vi "GetTempConfigByName.vi"(3 "Error In":errorcluster, 4 "JSON":string, 5 "Name":string) -> (0 "Error Out":errorcluster, 1 "Exist":bool, 2 "TempConfig":T1)   [LabVIEW 2014]
uses:
  TempConfig.ctl
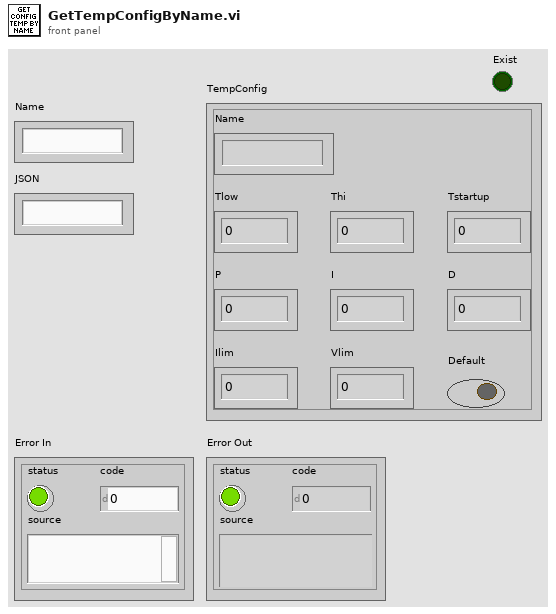
[diagram p1: front panel]
types:
  T1 = typedef "TempConfig.ctl" = cluster{"Name":string, "Thi":dbl, "Tlow":dbl, "Tstartup":dbl, "P":dbl, "I":dbl, "D":dbl, "Ilim":dbl, "Vlim":dbl, "Default":bool}
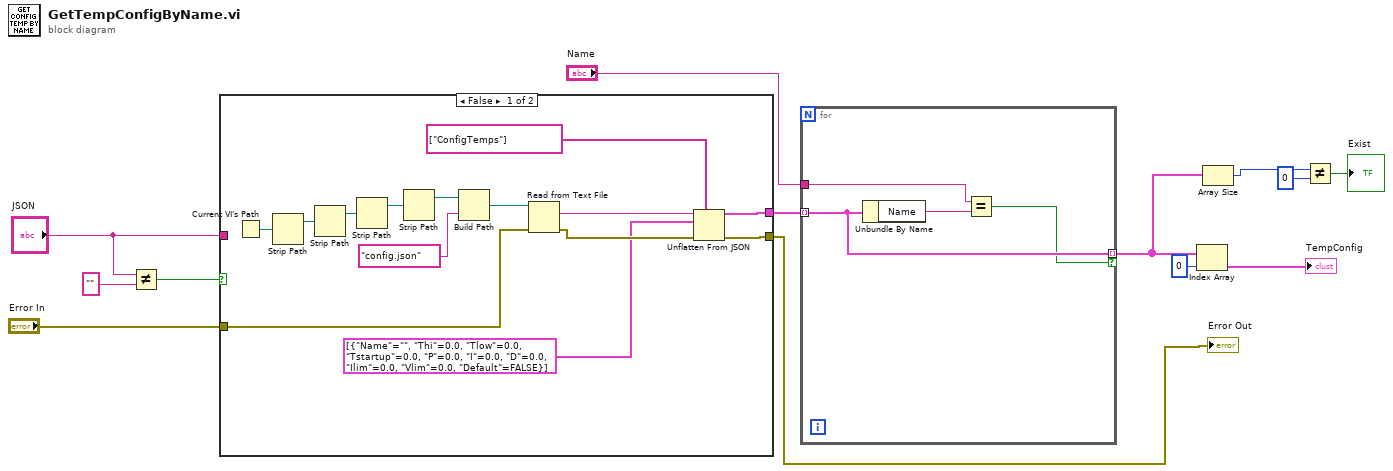
[diagram p0: block diagram]
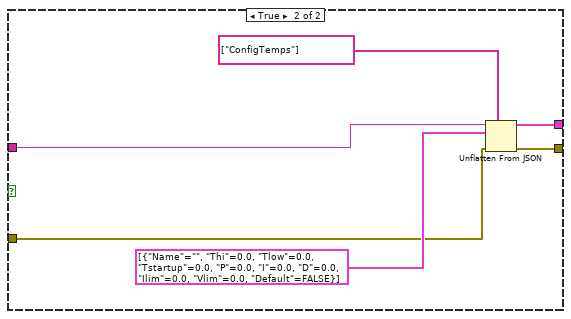
[diagram p2: hidden frame]
diagram:
  n1 = Not Equal?(x="JSON", y="") -> (x != y?=w6:bool)
  n2 = case shown="False" w6 {
    tunnel: [w16 w31] -> w13
    tunnel: [w15 w30] -> w10
    tunnel: "Error In" -> [w14 w29]
    tunnel: "JSON" -> [_ w28]
    frame False {
      n3 = Current VI's Path() -> (path=w17:path)
      n4 = Strip Path(path=w17) -> (stripped path=w21:path)  [unwired: 1 out]
      n5 = Strip Path(path=w21) -> (stripped path=w19:path)  [unwired: 1 out]
      n6 = Strip Path(path=w19) -> (stripped path=w20:path)  [unwired: 1 out]
      n7 = Strip Path(path=w20) -> (stripped path=w22:path)  [unwired: 1 out]
      n8 = Build Path(base path=w22, name or relative path="config.json") -> (appended path=w23:path)
      n9 = Read from Text File(file (use dialog)=w23, error in=w14) -> (text=w25:string, error out=w26:errorcluster)  [unwired: 2 in, 2 out]
      n10 = Unflatten From JSON(path=string[] ["ConfigTemps"], JSON string=w25, type and defaults=T1[] [{"Name"="", "Thi"=0.0, "Tlow"=0.0, "Tstartup"=0.0, "P"=0.0, "I"=0.0, "D"=0.0, "Ilim"=0.0, "Vlim"=0.0, "Default"=FALSE}], error in (no error)=w26) -> (value=w16:T1[], error out=w15:errorcluster)  [unwired: 3 in]
    }
    frame True {
      n11 = Unflatten From JSON(path=string[] ["ConfigTemps"], JSON string=w28, type and defaults=T1[] [{"Name"="", "Thi"=0.0, "Tlow"=0.0, "Tstartup"=0.0, "P"=0.0, "I"=0.0, "D"=0.0, "Ilim"=0.0, "Vlim"=0.0, "Default"=FALSE}], error in (no error)=w29) -> (value=w31:T1[], error out=w30:errorcluster)  [unwired: 3 in]
    }
  }
  "Error Out" <- w10
  n12 = for {
    tunnel: w13 -> [w35] mode=indexing
    tunnel: "Name" -> [w36]
    tunnel: [w35] -> w4 mode=indexing if=w34
    n13 = Unbundle By Name(w35) -> ("Name"=w37:string)
    n14 = Equal?(x=w36, y=w37) -> (x = y?=w34:bool)
  }
  n15 = Index Array(array=w4, index=0) -> (element=→"TempConfig":T1)
  n16 = Array Size(array=w4) -> (size(s)=w3:i32)
  n17 = Not Equal?(x=w3, y=0) -> (x != y?=→"Exist":bool)
